vi "value2range_AAC.vi"(2 "Current [A]":dbl) -> (1 "Limited current [A]":dbl, 4 "Positive or zero":bool, 6 "Range limit [A]":dbl, 7 "Range [-]":i32, 8 "Positive":bool, 9 "Overflow":bool)   [LabVIEW 2020, in "Datron D4xxx.lvlib"]
doc: "This VI returns range code for entered current."
uses:
  Datron D4xxx.lvlib
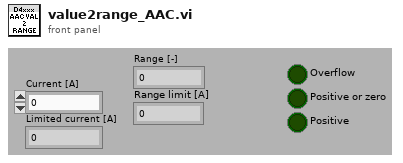
[diagram p1: front panel]
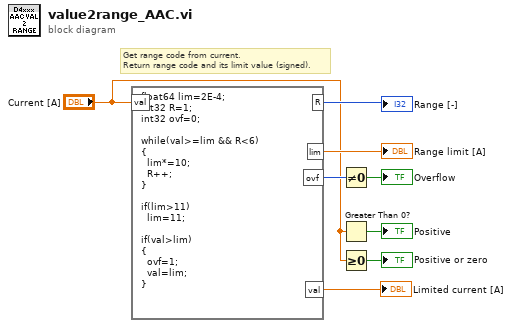
[diagram p0: block diagram]
diagram:
  # "Get range code from current.\nReturn range code and its limit value (signed)."
  n1 = formula code="float64 lim=2E-4;\nint32 R=1;\nint32 ovf=0;\n\nwhile(val>=lim && R<6)\n{\n  lim*=10;\n  R++;\n}\n\nif(lim>11)\n  lim=11;\n\nif(val>lim)\n{\n  ovf=1;\n  val=lim;\n}"("val"="Current [A]") -> ("R"=→"Range [-]":i32, "lim"=→"Range limit [A]":dbl, "ovf"=w6:i32, "val"=→"Limited current [A]":dbl)
  n2 = Not Equal To 0?(x=w6) -> (x != 0?=→"Overflow":bool)
  n3 = Greater Than 0?(x="Current [A]") -> (x > 0?=→"Positive":bool)
  n4 = Greater Or Equal To 0?(x="Current [A]") -> (x >= 0?=→"Positive or zero":bool)
